vi "ConnectSalicruAPI (SubVI).vi"(8 "error in (no error)":errorcluster, 10 "SALICRU WRAPPER FILE":path, 11 "Refnum in":refnum<k35>) -> (0 "error out":errorcluster, 3 "Refnum out":refnum<k35>)   [LabVIEW 2024, in "SALICRUAPI.lvlib"]
uses:
  SALICRUAPI.lvlib
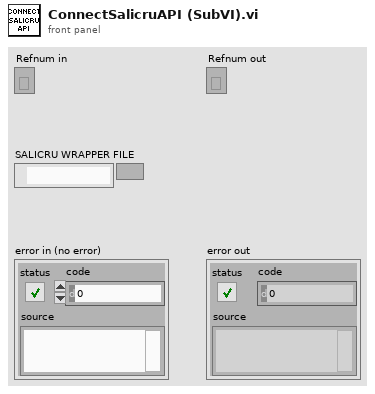
[diagram p1: front panel]
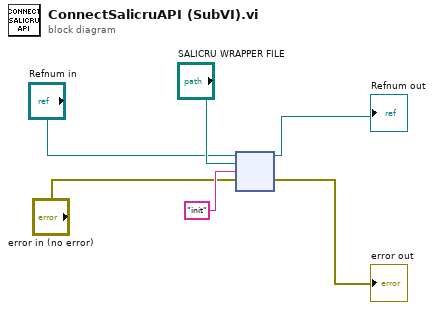
[diagram p0: block diagram]
diagram:
  n1 = node("Refnum in", "SALICRU WRAPPER FILE", "init" ("function name"), "error in (no error)") -> (→"Refnum out":refnum<k35>, →"error out":errorcluster)  [unwired: 2 in, 2 out]
